vi "Get Model Number.vi"(8 "error in":errorcluster, 11 "Alicat Device in":refnum<class "Alicat Device.lvclass">=refnum) -> (0 "error out":errorcluster, 2 "DataOut":string, 3 "Alicat Device out":refnum<class "Alicat Device.lvclass">)   [LabVIEW 2014]
uses:
  reusable/Session APIs/Serial/Serial Session.lvclass
  reusable/Session APIs/Serial/Public/Get Data/Get String.vi
  Alicat Device.lvclass
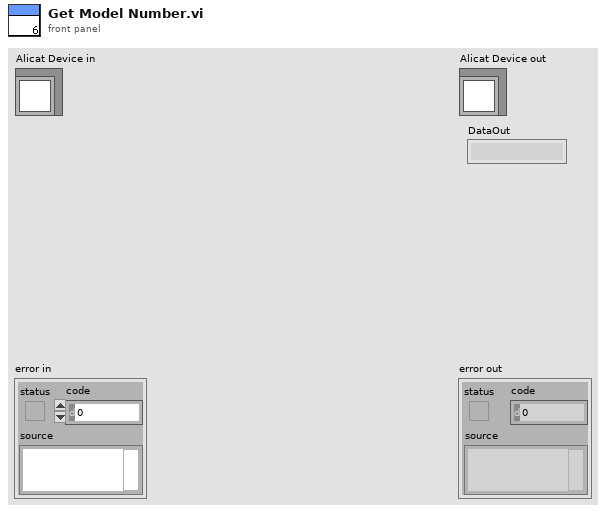
[diagram p1: front panel]
types:
  T1 = typedef "Serial Session.lvclass/Session Handle.ctl" = refnum<data-value>
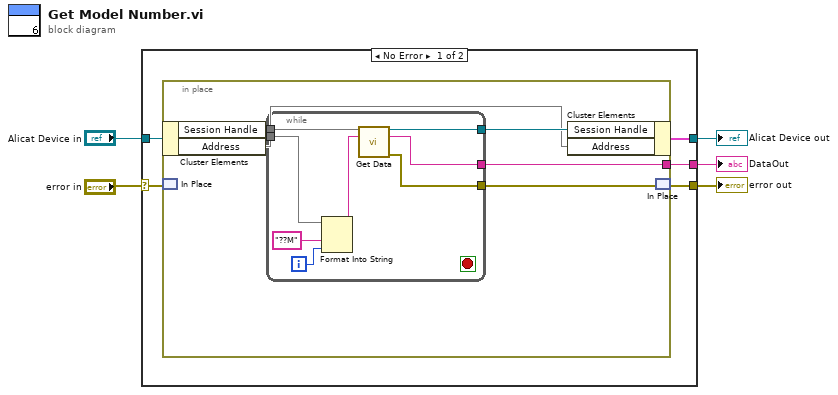
[diagram p0: block diagram]
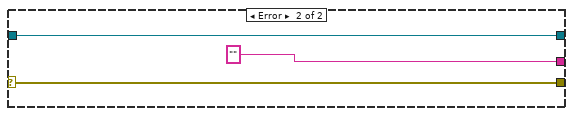
[diagram p2: hidden frame]
diagram:
  n1 = case shown="No Error" "error in" {
    selector: "error in" -> [w9 w26]
    tunnel: "Alicat Device in" -> [w10 w25]
    tunnel: [w7 w26] -> w1
    tunnel: [w8 w25] -> w3
    tunnel: [w6 "" ("DataOut")] -> w4
    frame No Error {
      n2 = in-place {
        in-place-border: [w12] -> w6
        n3 = in-place-cluster #1(w10) -> ("Session Handle"=w15, "Address"=w11)
        n4 = in-place-match #2(w9) -> ()  [unwired: 1 out]
        n5 = while {
          tunnel: w15 -> [w23]
          tunnel: [w22] -> w14
          tunnel: [w21] -> w13
          tunnel: [w20] -> w12
          tunnel: w11 -> [w18]
          i -> [w19]
          stop <- _ stop-if-true
          n6 = Format Into String(initial string=w18, "??M" ("Address"), w19) -> (resulting string=w16:string)  [unwired: 2 in, 1 out]
          n7 = call-poly "Get Data.vi"("Session Handle in"=w23, "CMD"=w16) -> ("Session Handle out"=w22:T1, "DataOut"=w20:string, "error out"=w21:errorcluster)  [unwired: 11 in]
        }
        n8 = in-place-cluster #1("Session Handle"=w14, "Address"=w11) -> (w8:cluster{})
        n9 = in-place-match #2(w13) -> (w7:errorcluster)
      }
    }
    frame Error {
    }
  }
  "error out" <- w1
  "Alicat Device out" <- w3
  "DataOut" <- w4
